vi "customOp_compBasicSwitch.vi"(10 "Channel":T1={"Operation"=0, "Input A"=0, "Output - LO"=0.0, "Output - HI"=0.0, "Inputs"=[0, 0, 0, 0], "Output Values"=[0.0, 0.0, 0.0, 0.0, 0.0], "Num. Inputs"=4, "Set Point"=0.0, "Inv."=[FALSE, FALSE, FALSE, FALSE], "Inv. A"=FALSE, "Inv. B"=FALSE, "Input B"=0} {"Input B" items=["DIO0", "DIO1", "DIO2", "DIO3", "DIO4", "DIO5", "DIO6", "DIO7", "DIO8", "DIO9", "DIO10", "DIO11", "DIO12", "DIO13", "DIO14", "DIO15", "DIO16", "DIO17", "DIO18", "DIO19", "DIO20", "DIO21", "DIO22", "DIO23", "DIO24", "DIO25", "DIO26", "DIO27", "DIO28", "DIO29", "DIO30", "DIO31", "FALSE"]; "Input A" items=["DIO0", "DIO1", "DIO2", "DIO3", "DIO4", "DIO5", "DIO6", "DIO7", "DIO8", "DIO9", "DIO10", "DIO11", "DIO12", "DIO13", "DIO14", "DIO15", "DIO16", "DIO17", "DIO18", "DIO19", "DIO20", "DIO21", "DIO22", "DIO23", "DIO24", "DIO25", "DIO26", "DIO27", "DIO28", "DIO29", "DIO30", "DIO31", "FALSE"]; "Inputs" items=["DIO0", "DIO1", "DIO2", "DIO3", "DIO4", "DIO5", "DIO6", "DIO7", "DIO8", "DIO9", "DIO10", "DIO11", "DIO12", "DIO13", "DIO14", "DIO15", "DIO16", "DIO17", "DIO18", "DIO19", "DIO20", "DIO21", "DIO22", "DIO23", "DIO24", "DIO25", "DIO26", "DIO27", "DIO28", "DIO29", "DIO30", "DIO31", "FALSE"]; "Operation" items=["OFF", "Constant", "Bool - Basic Switch", "Bool - AND Switch", "Bool - OR Switch", "Custom - Comp Basic Switch", "Custom - 461nm Freq."]}, 11 "Digital Input Value Array":bool[](array[boolean])=[FALSE, FALSE, FALSE, FALSE, FALSE, FALSE, FALSE, FALSE, FALSE, FALSE, FALSE, FALSE, FALSE, FALSE, FALSE, FALSE, FALSE, FALSE, FALSE, FALSE, FALSE, FALSE, FALSE, FALSE, FALSE, FALSE, FALSE, FALSE, FALSE, FALSE, FALSE, FALSE]) -> (3 "AO Out":fxp<+/-,20,5>)   [LabVIEW 2016]
uses:
  op_ctrl_element.ctl
  DIO_selector.ctl
  output_value.ctl
panel:
  # "Constant Operation Control"
  # "Boolean Operation Control"
  # "Custom Operation Controls"
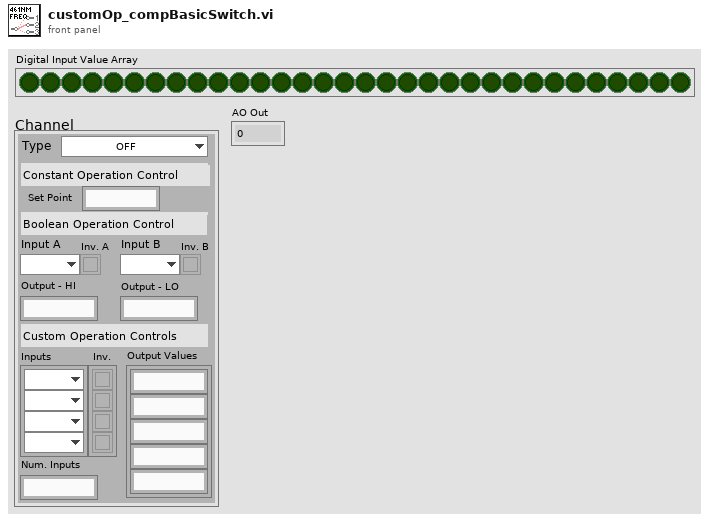
[diagram p1: front panel]
types:
  T1 = typedef "op_ctrl_element.ctl" = cluster{"Operation":i16, "Input A":T2, "Output - LO":T3, "Output - HI":T3, "Inputs":T2[], "Output Values":T3[], "Num. Inputs":i32, "Set Point":T3, "Inv.":bool[], "Inv. A":bool, "Inv. B":bool, "Input B":T2}
  T2 = typedef "DIO_selector.ctl" = i32
  T3 = typedef "output_value.ctl" = fxp<+/-,20,5>
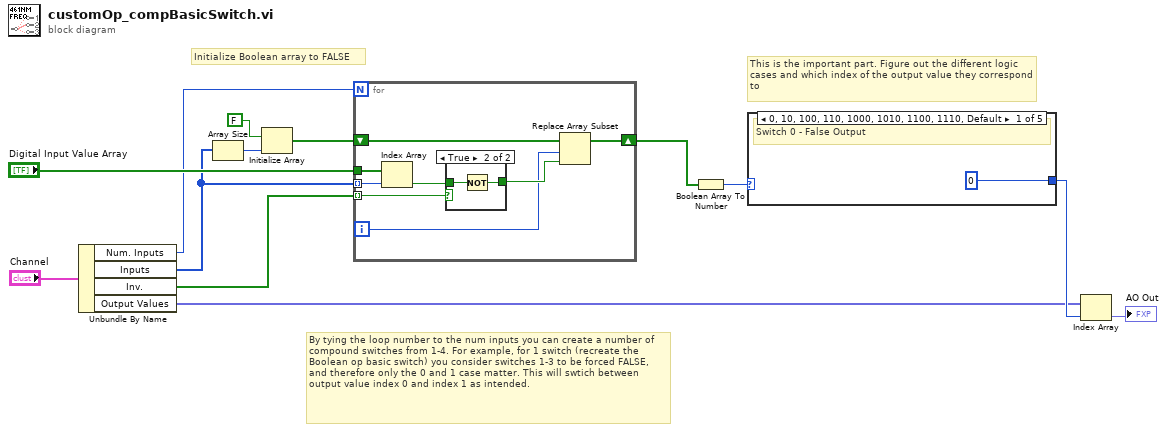
[diagram p0: block diagram]
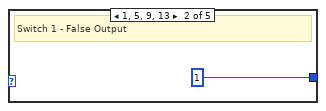
[diagram p2: hidden frame]
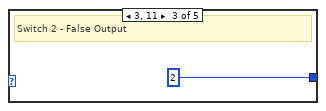
[diagram p3: hidden frame]
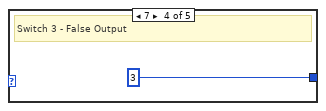
[diagram p4: hidden frame]
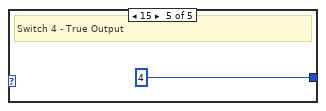
[diagram p5: hidden frame]
diagram:
  # "By tying the loop number to the num inputs you can create a number of compound switches from 1-4. For example, for 1 switch (recreate the Boolean op basic switch) you consider switches 1-3 to be forced FALSE, and therefore only the 0 and 1 case matter. This will swtich between output value index 0 and index 1 as intended."
  # "This is the important part. Figure out the different logic cases and which index of the output value they correspond to"
  # "Initialize Boolean array to FALSE"
  n1 = Unbundle By Name("Channel") -> ("Num. Inputs"=w3:i32, "Inputs"=w8:T2[], "Inv."=w1:bool[], "Output Values"=w2:T3[])
  n2 = Array Size(array=w8) -> (size(s)=w7:i32)
  n3 = Initialize Array(FALSE, w7) -> (w5:bool[])
  n4 = for {
    N: w3 -> [_]
    tunnel: "Digital Input Value Array" -> [w21]
    tunnel: w8 -> [w20] mode=indexing
    shift-right: [w17] -> w4
    shift-left: w5 -> [w14]
    tunnel: w1 -> [w19] mode=indexing
    i -> [w15]
    n5 = Index Array(array=w21, index=w20) -> (element=w18:bool)
    n6 = case shown="True" w19 {
      tunnel: w18 -> [w22 w24]
      tunnel: [w22 w23] -> w16
      frame False {
      }
      frame True {
        n7 = Not(x=w24) -> (.not. x?=w23:bool)
      }
    }
    n8 = Replace Array Subset(array=w14, new element=w16, index=w15) -> (w17:bool[])
  }
  n9 = Boolean Array To Number(Boolean array=w4) -> (number=w11:u32)
  n10 = case shown="0, 10, 100, 110, 1000, 1010, 1100, 1110, Default" w11 {
    tunnel: [0 1 2 3 4] -> w10
    frame 0, 2, 4, 6, 8, 10, 12, 14, Default {
      # "Switch 0 - False Output"
    }
    frame 1, 5, 9, 13 {
      # "Switch 1 - False Output"
    }
    frame 3, 11 {
      # "Switch 2 - False Output"
    }
    frame 7 {
      # "Switch 3 - False Output"
    }
    frame 15 {
      # "Switch 4 - True Output"
    }
  }
  n11 = Index Array(array=w2, index=w10) -> (element=→"AO Out":T3)
